vi "Replace Array Elements [DBL].vi"(8 "Error In":errorcluster, 9 "Array of Replacement Pairs":cluster{"Original":dbl, "New":dbl}[](array[cluster]), 11 "Array":dbl[](array[numeric])) -> (0 "Error Out":errorcluster, 3 "Array with Replacements":dbl[](array[numeric]))   [LabVIEW 2021, in "Arrays.lvlib"]
uses:
  Arrays.lvlib
  <userlib>/_OpenG.lib/array/array.llb/Search 1D Array (DBL)__ogtk.vi
  <userlib>/_OpenG.lib/array/array.llb/openg_array.lvlib
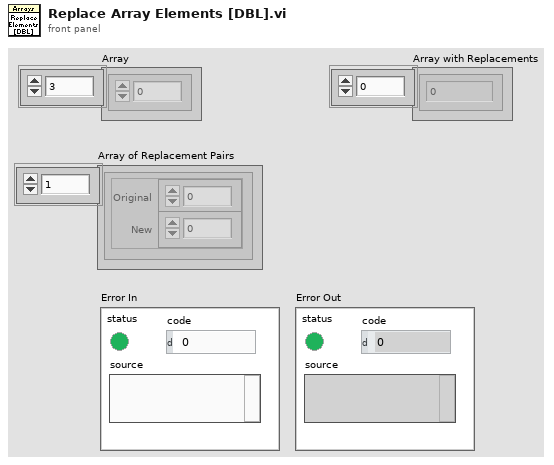
[diagram p1: front panel]
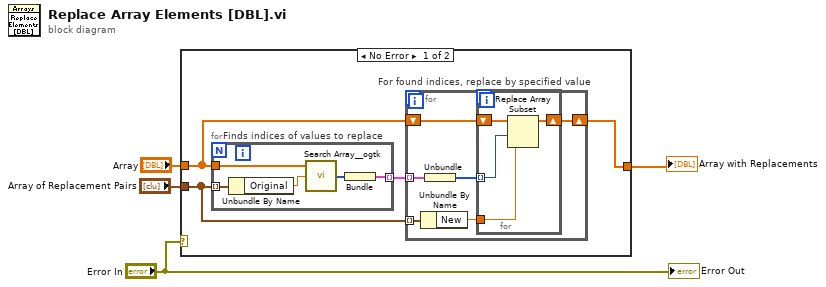
[diagram p0: block diagram]
diagram:
  n1 = case shown="No Error" "Error In" {
    tunnel: "Array" -> [w8 w24]
    tunnel: "Array of Replacement Pairs" -> [w6 _]
    tunnel: [w5 w24] -> w2
    frame No Error {
      n2 = for "Finds indices of values to replace" {
        tunnel: w6 -> [w22] mode=indexing
        tunnel: w8 -> [w23]
        tunnel: [w19] -> w7 mode=indexing
        n3 = Unbundle By Name(w22) -> ("Original"=w21:dbl)
        n4 = call-poly <userlib>:"Search Array__ogtk.vi"("Array"=w23, "Element Data"=w21) -> ("Indices of Elements"=w20:i32[])  [unwired: 7 in]
        n5 = Bundle("Indices of Elements"=w20) -> (w19:cluster{"Indices of Elements":i32[]})  [unwired: 1 in]
      }
      n6 = for "For found indices, replace by specified value" {
        tunnel: w6 -> [w14] mode=indexing
        tunnel: w7 -> [w13] mode=indexing
        shift-right: [w11] -> w5
        shift-left: w8 -> [w12]
        n7 = Unbundle By Name(w14) -> ("New"=w9:dbl)
        n8 = Unbundle(w13) -> ("Indices of Elements"=w10:i32[])
        n9 = for {
          shift-right: [w15] -> w11
          shift-left: w12 -> [w18]
          tunnel: w10 -> [w17] mode=indexing
          tunnel: w9 -> [w16]
          n10 = Replace Array Subset(array=w18, new element=w16, index=w17) -> (w15:dbl[])
        }
      }
    }
    frame Error {
    }
  }
  "Array with Replacements" <- w2
  "Error Out" <- "Error In"
